vi "Traverse_Space.vi"(9 "Show Panel?":bool, 10 "Traverse Setup":string) -> (3 "Error Comments":string)   [LabVIEW 2011]
doc: "This is an example of using features of the VI Server as a client. It shows how you might browse from one or more applications that may be exporting data from one or more data stations. \n\nThe example shows how to query a server for its list of exported VIs, how to get references to the VIs, and how call them with the Call By Reference function."
uses:
  Route mapping/Exclude_cluster.ctl
  Route mapping/Box_size.ctl
  Route mapping/Exclusion_type.ctl
  Controls/ok_button.ctl
  Globals/Constants_global.vi
  Route mapping/Route_mapping_global.vi
  Globals/Trav_pos_global.vi
panel:
  in  "Traverse space filename":u16(ring) items=["Default_Space_file.xls", "---Save As---"]
  in  "Traverse Name":u16(ring) items=["A_Tunnel"]
  out "Message":string
  in  "Cancel Button":bool
  in  "OK":T1
  in  "Entire Space":T2=[{"Max"=15001.0, "Min"=12000.0}, {"Max"=1000.0, "Min"=-1000.0}, {"Max"=700.0, "Min"=0.0}] {"Min" format="%#.1f"; "Max" format="%#.1f"}
  in  "Probe Volume":T2=[{"Max"=15.0, "Min"=-15.0}, {"Max"=250.0, "Min"=0.0}, {"Max"=15.0, "Min"=-15.0}] {"Min" format="%#.1f"; "Max" format="%#.1f"}
  in  "Exclude Array":T3[](array[typedef])=[{"Sizes"=[{"Max"=15000.0, "Min"=0.0}, {"Max"=1000.0, "Min"=-1000.0}, {"Max"=300.0, "Min"=0.0}], "Name"="Roughness Elements", "Exclude Type"=enum."Allow only vertical moves"}, {"Sizes"=[{"Max"=17000.0, "Min"=16000.0}, {"Max"=200.0, "Min"=-200.0}, {"Max"=-50.0, "Min"=-250.0}], "Name"="B204", "Exclude Type"=enum."Exclude completely"}] {"Sizes"."Min" format="%#.1f"; "Sizes"."Max" format="%#.1f"}
  # "Enter all coordinates assuming the Model Orientation is zero degrees"
  # "(Relative to measurement position)"
  # "X                           Y                          Z"
  # "X                           Y                          Z"
  # "(Relative to measurement position)"
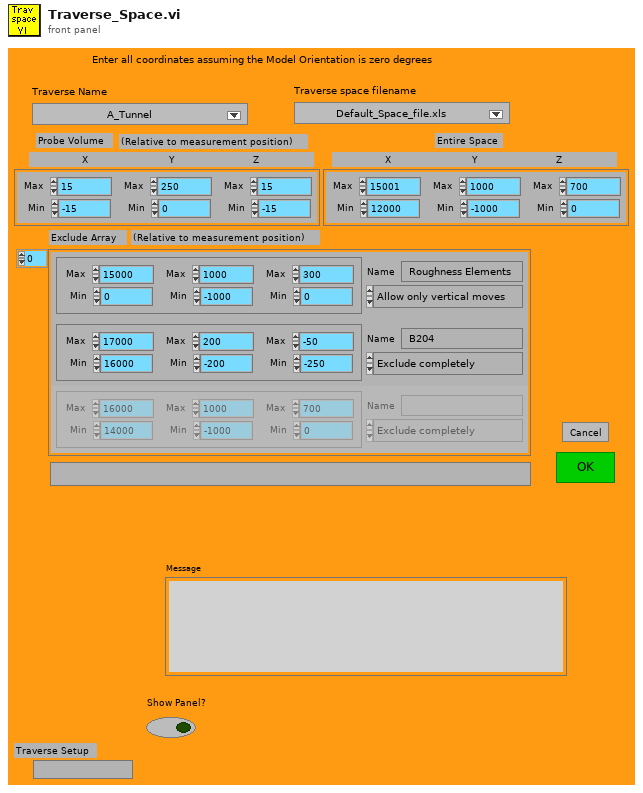
[diagram p1: front panel]
types:
  T1 = typedef "ok_button.ctl" = bool
  T2 = typedef "Box_size.ctl" = cluster{"Max":dbl, "Min":dbl}[]
  T3 = typedef "Exclude_cluster.ctl" = cluster{"Sizes":T2, "Name":string, "Exclude Type":T4}
  T4 = typedef "Exclusion_type.ctl" = enum16{"Exclude completely", "Allow only vertical moves"}
  T5 = enum16{"Load setup from excel file", "Save setup to excel file"}
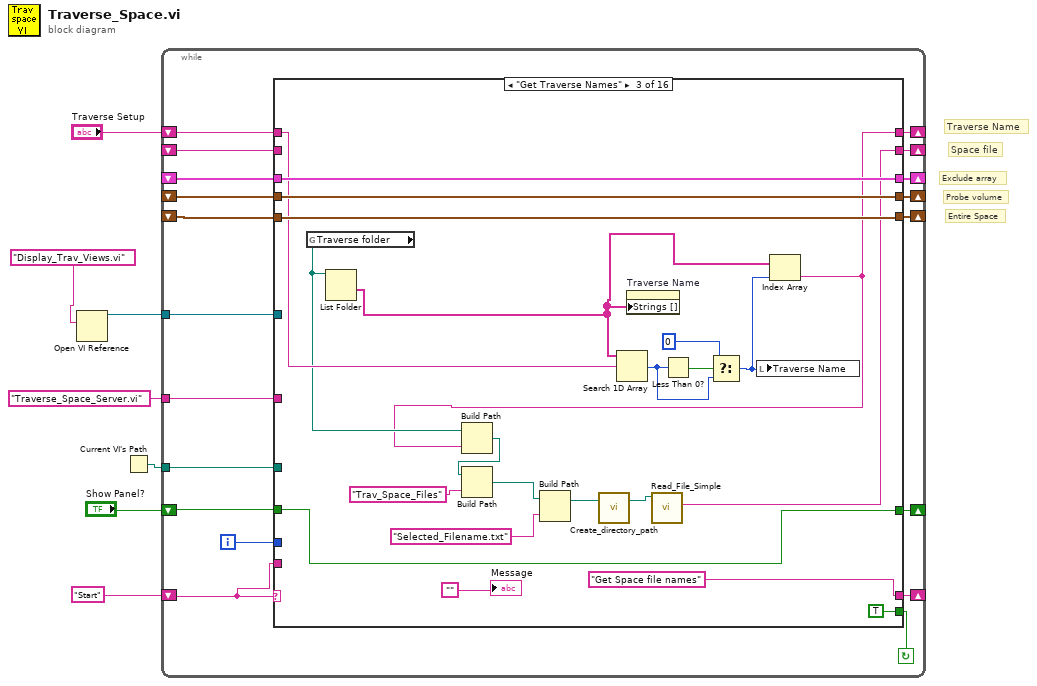
[diagram p0: block diagram]
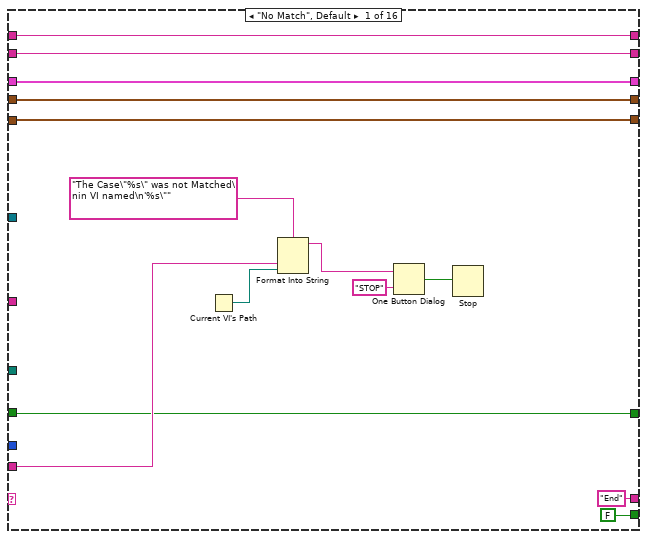
[diagram p2: hidden frame]
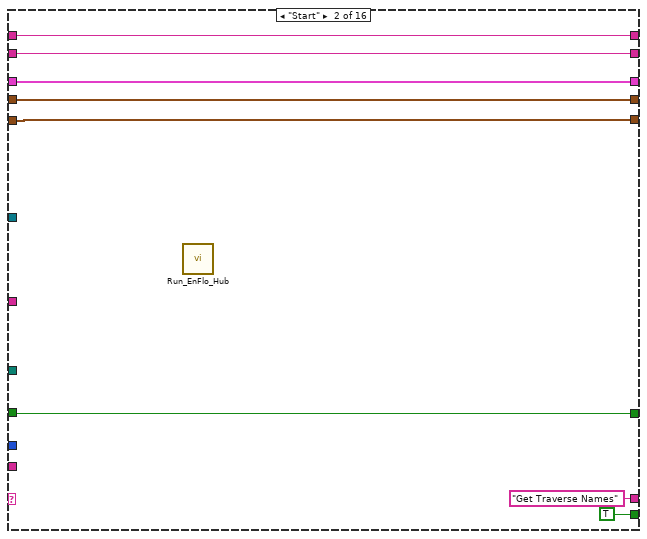
[diagram p3: hidden frame]
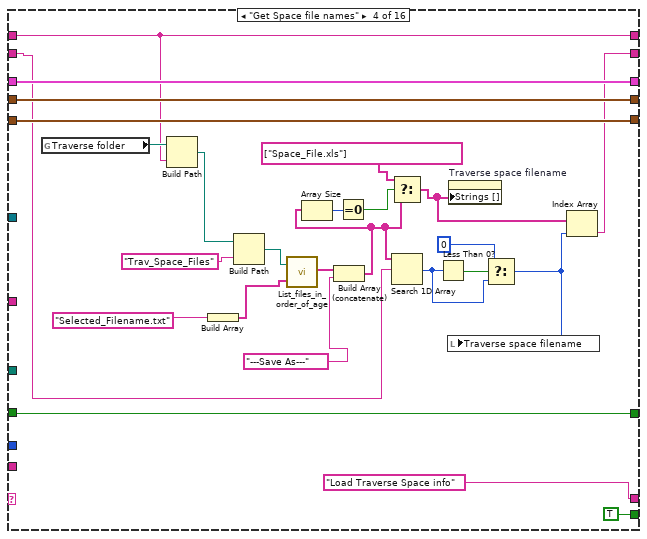
[diagram p4: hidden frame]
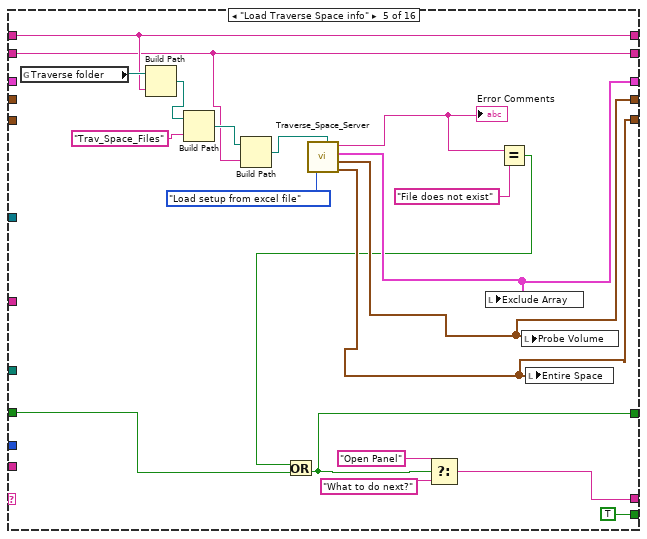
[diagram p5: hidden frame]
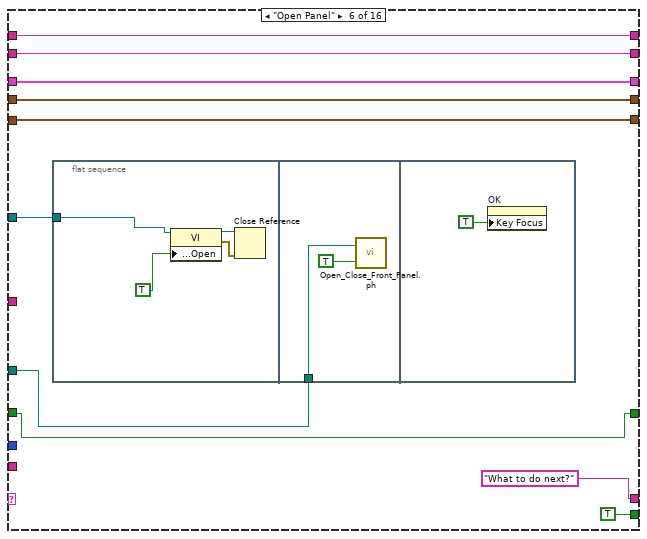
[diagram p6: hidden frame]
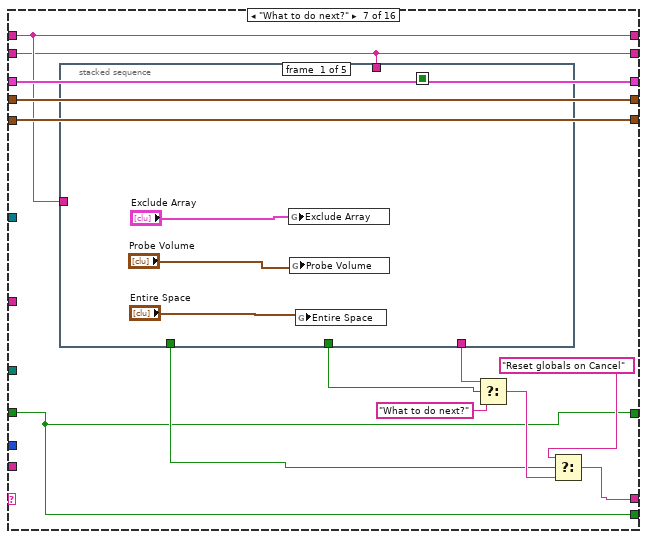
[diagram p7: hidden frame]
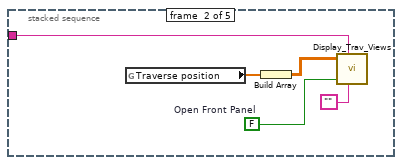
[diagram p8: hidden frame]
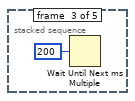
[diagram p9: hidden frame]
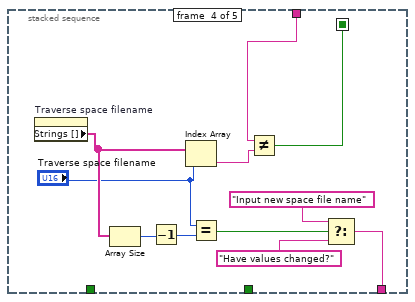
[diagram p10: hidden frame]
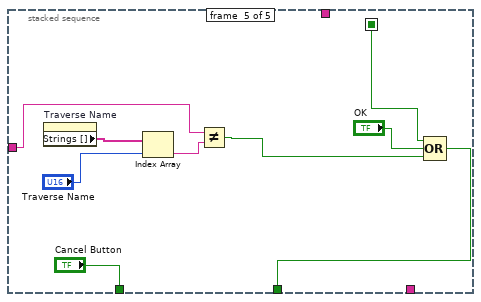
[diagram p11: hidden frame]
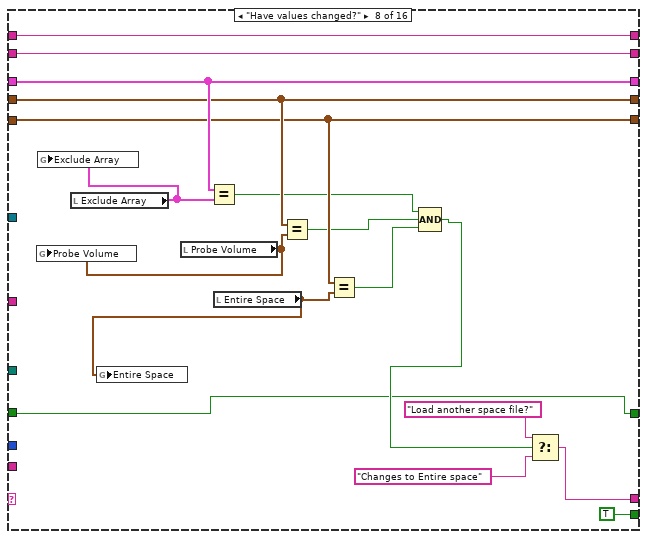
[diagram p12: hidden frame]
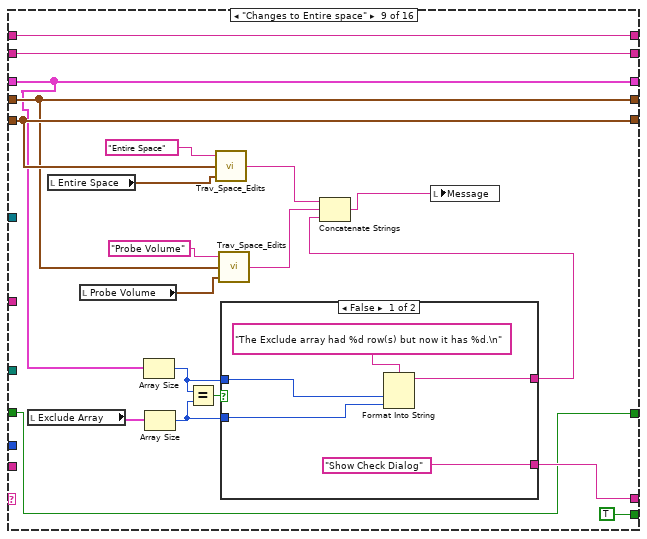
[diagram p13: hidden frame]
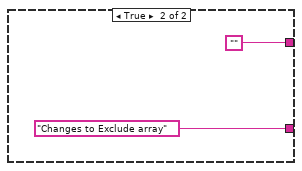
[diagram p14: hidden frame]
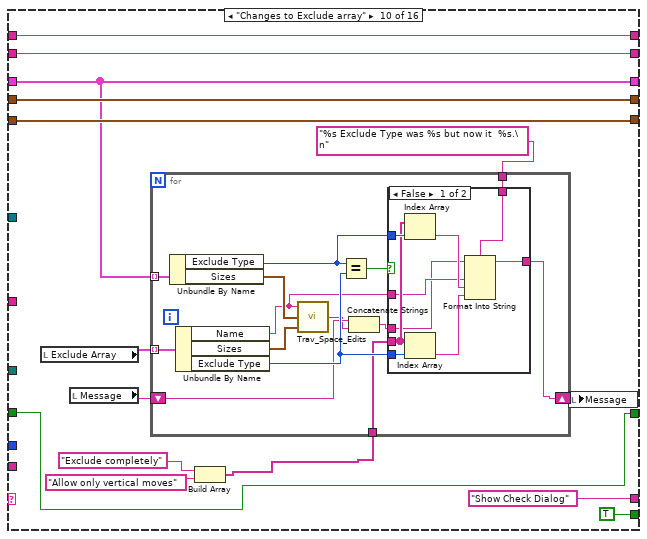
[diagram p15: hidden frame]
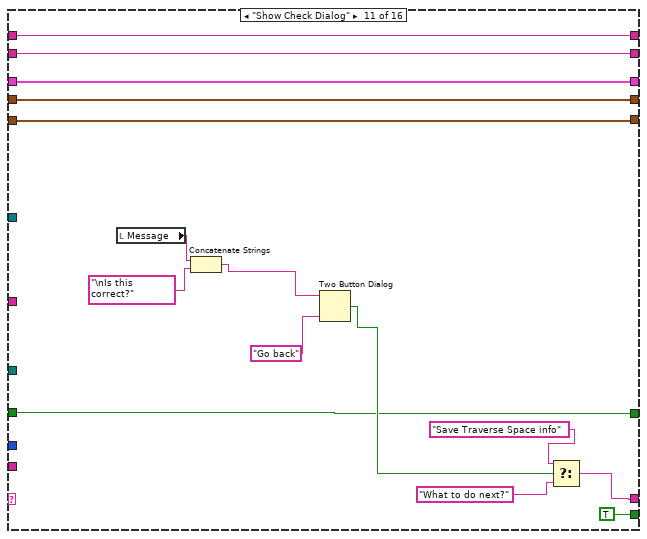
[diagram p17: hidden frame]
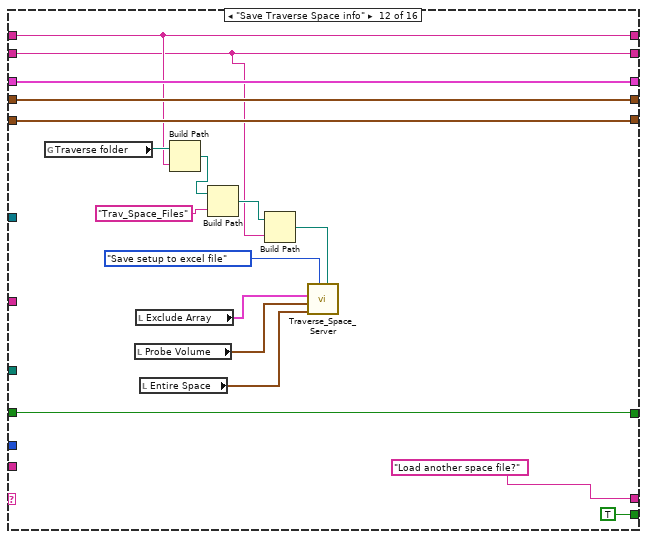
[diagram p18: hidden frame]
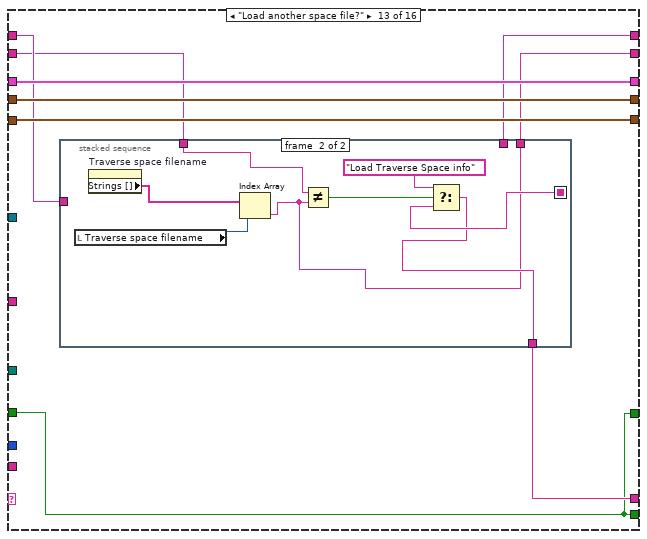
[diagram p19: hidden frame]
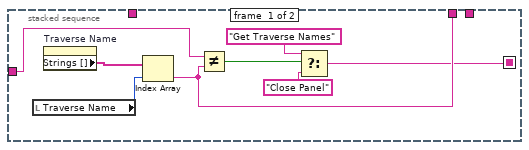
[diagram p20: hidden frame]
diagram:
  # "Traverse Name"
  # "Space file"
  # "Entire Space"
  # "Probe volume"
  # "Exclude array"
  n1 = Open VI Reference(vi path="Display_Trav_Views.vi") -> (vi reference=w1:refnum<vi>)  [unwired: 1 in, 5 out]
  n2 = Current VI's Path() -> (path=w5:path)
  n3 = while {
    tunnel: "Traverse_Space_Server.vi" ("VI name to run on server") -> [w24]
    shift-left: "Start" -> [w21]
    shift-right: [w23] -> _
    tunnel: w5 -> [w22]
    shift-right: [w20] -> _
    shift-left: _ -> [w17]
    shift-right: [w19] -> _
    shift-left: _ -> [w16]
    shift-right: [w18] -> _
    shift-left: _ -> [w15]
    shift-right: [w13] -> _
    shift-left: "Traverse Setup" -> [w11]
    shift-right: [w14] -> _
    shift-left: _ -> [w12]
    shift-right: [w9] -> _
    shift-left: "Show Panel?" -> [w10]
    tunnel: w1 -> [w8]
    i -> [w26]
    stop <- w25 continue-if-true
    n4 = case shown="\"Get Traverse Names\"" w21 {
      tunnel: w26 -> [_ _ _ _ _ _ _ _ _ _ _ _ _ _ _ _]
      tunnel: [FALSE ("status") TRUE ("status") TRUE ("status") TRUE ("status") TRUE ("status") TRUE ("status") w134 TRUE ("status") TRUE ("status") TRUE ("status") TRUE ("status") TRUE ("status") w291 w316 TRUE ("status") FALSE ("status")] -> w25
      tunnel: ["End" ("f") "Get Traverse Names" ("f") "Get Space file names" "Load Traverse Space info" w115 "What to do next?" w145 w182 w200 "Show Check Dialog" ("f") w263 "Load another space file?" w292 w317 "Close Panel" "End"] -> w23
      tunnel: w24 -> [_ _ _ _ _ _ _ _ _ _ _ _ _ _ _ _]
      tunnel: w10 -> [w27 w41 w49 w71 w99 w118 w134 w179 w193 w220 w259 w274 w291 w316 w340 w352]
      tunnel: w22 -> [_ _ _ _ _ w121 _ _ _ _ _ _ _ _ _ w366]
      tunnel: w21 -> [w35 _ _ _ _ _ _ _ _ _ _ _ _ _ _ _]
      tunnel: [w32 w48 w68 w94 w114 w124 w143 w192 w203 w230 w273 w288 w299 w327 w346 w365] -> w20
      tunnel: [w31 w47 w67 w93 w113 w123 w142 w191 w206 w232 w272 w287 w298 w326 w345 w364] -> w19
      tunnel: [w30 w46 w66 w92 w112 w122 w141 w190 w210 w233 w270 w286 w297 w325 w344 w363] -> w18
      tunnel: w17 -> [w32 w48 w68 w94 _ w124 w143 w192 w203 w230 w273 w288 w299 w327 w346 w365]
      tunnel: w16 -> [w31 w47 w67 w93 _ w123 w142 w191 w206 w232 w272 w287 w298 w326 w345 w364]
      tunnel: w15 -> [w30 w46 w66 w92 _ w122 w141 w190 w210 w233 w270 w286 w297 w325 w344 w363]
      tunnel: [w28 w42 w51 w77 w103 w119 w137 w180 w194 w221 w260 w276 w293 w320 w341 w353] -> w14
      tunnel: [w29 w43 w57 w76 w107 w120 w138 w181 w195 w222 w261 w277 w295 w324 w342 w358] -> w13
      tunnel: w12 -> [w28 w42 _ w75 w103 w119 w137 w180 w194 w221 w260 w276 w294 w319 w341 w353]
      tunnel: w11 -> [w29 w43 w60 w76 w107 w120 w138 w181 w195 w222 w261 w277 w296 w324 w342 w358]
      tunnel: [w27 w41 w49 w71 w97 w118 w134 w179 w193 w220 w259 w274 w291 w316 w340 w352] -> w9
      tunnel: w8 -> [_ _ _ _ _ w117 _ _ _ _ _ _ _ _ _ w348]
      frame "No Match", Default {
        n5 = Current VI's Path() -> (path=w40:path)
        n6 = Format Into String(format string="The Case\"%s\" was not Matched\nin VI named\n'%s\"" ("Format String"), w35, w40) -> (resulting string=w37:string)  [unwired: 2 in, 1 out]
        n7 = One Button Dialog(message=w37, button name ("OK")="STOP") -> (true=w39:bool)
        n8 = Stop(stop? (T)=w39) -> ()
      }
      frame "Start" {
        n9 = call "Run_EnFlo_Hub.vi"() -> ()  [unwired: 8 out]
      }
      frame "Get Traverse Names" {
        n10 = global read "Constants_global.vi" "Traverse folder"() -> (w58:path)
        n11 = List Folder(path=w58) -> (folder names=w50:string[])  [unwired: 1 in, 5 out]
        n12 = Search 1D Array(1D array=w50, element=w60) -> (index of element=w63:i32)  [unwired: 1 out]
        n13 = property on="Traverse Name" class="Ring (strict)"("Strings []"=w50) -> ()  [unwired: 2 in, 2 out]
        n14 = Less Than 0?(x=w63) -> (x < 0?=w64:bool)
        n15 = Select(t=0, s=w64, f=w63) -> (s? t:f=w61:i32)
        n16 = local write "Traverse Name"(w61) -> ()
        n17 = Index Array(array=w50, index=w61) -> (element=w57:string)
        n18 = Build Path(base path=w58, name or relative path=w57) -> (appended path=w56:path)
        n19 = Build Path(base path=w56, name or relative path="Trav_Space_Files" ("Substring")) -> (appended path=w55:path)
        n20 = Build Path(base path=w55, name or relative path="Selected_Filename.txt" ("Substring")) -> (appended path=w52:path)
        n21 = call "Create_directory_path.vi"("Path name"=w52) -> ("Path name Out"=w53:path)  [unwired: 1 in, 1 out]
        n22 = call "Read_File_Simple.vi"("Filename"=w53) -> ("string"=w51:string)  [unwired: 2 in, 7 out]
        "Message" <- ""
      }
      frame "Get Space file names" {
        n23 = global read "Constants_global.vi" "Traverse folder"() -> (w88:path)
        n24 = Build Path(base path=w88, name or relative path=w76) -> (appended path=w86:path)
        n25 = Build Array("Selected_Filename.txt" ("Substring")) -> (w85:string[])
        n26 = Build Path(base path=w86, name or relative path="Trav_Space_Files" ("Substring")) -> (appended path=w78:path)
        n27 = call "List_files_in_order_of_age.vi"("Files to Hide"=w85, "Folder"=w78) -> ("file names"=w74:string[])
        n28 = Build Array (concatenate)(w74, "---Save As---") -> (w73:string[])
        n29 = Array Size(array=w73) -> (size(s)=w83:i32)
        n30 = Equal To 0?(x=w83) -> (x = 0?=w82:bool)
        n31 = Select(t=string[] ["Space_File.xls"] ("appended array"), s=w82, f=w73) -> (s? t:f=w80:string[])
        n32 = Search 1D Array(1D array=w73, element=w75) -> (index of element=w90:i32)  [unwired: 1 out]
        n33 = Less Than 0?(x=w90) -> (x < 0?=w91:bool)
        n34 = property on="Traverse space filename" class="Ring (strict)"("Strings []"=w80) -> ()  [unwired: 2 in, 2 out]
        n35 = Select(t=0, s=w91, f=w90) -> (s? t:f=w79:i32)
        n36 = local write "Traverse space filename"(w79) -> ()
        n37 = Index Array(array=w80, index=w79) -> (element=w77:string)
      }
      frame "Load Traverse Space info" {
        n38 = global read "Constants_global.vi" "Traverse folder"() -> (w108:path)
        n39 = Build Path(base path=w108, name or relative path=w107) -> (appended path=w105:path)
        n40 = Build Path(base path=w105, name or relative path="Trav_Space_Files" ("Substring")) -> (appended path=w104:path)
        n41 = Build Path(base path=w104, name or relative path=w103) -> (appended path=w102:path)
        n42 = call "Traverse_Space_Server.vi"("Space File"=w102, "Mode"=T5."Load setup from excel file") -> ("Entire Space Out"=w112:T2, "Probe Volume Out"=w113:T2, "Exclude Array Out"=w114:T3[], "Error Comments"=w100:string)  [unwired: 5 in]
        "Error Comments" <- w100
        n43 = local write "Exclude Array"(w114) -> ()
        n44 = Equal?(x=w100, y="File does not exist") -> (x = y?=w98:bool)
        n45 = Or(x=w98, y=w99) -> (x .or. y?=w97:bool)
        n46 = Select(t="Open Panel", s=w97, f="What to do next?") -> (s? t:f=w115:string)
        n47 = local write "Probe Volume"(w113) -> ()
        n48 = local write "Entire Space"(w112) -> ()
      }
      frame "Open Panel" {
        n49 = flat-sequence {
          tunnel: w117 -> [w127]
          tunnel: w121 -> [w131]
          frame #0 {
            n50 = property class="VI"(reference=w127, "Front Panel Window:Open"=TRUE) -> (reference out=w129:refnum<vi>, error out=w128:errorcluster)  [unwired: 1 in]
            n51 = Close Reference(reference=w129, error in (no error)=w128) -> ()  [unwired: 1 out]
          }
          frame #1 {
            n52 = call "Open_Close_Front_Panel.ph.vi"("Front Panel Window:Open"=TRUE, "VI path"=w131) -> ()  [unwired: 2 out]
          }
          frame #2 {
            n53 = property on="OK" class="Bool"("Key Focus"=TRUE) -> ()  [unwired: 2 in, 2 out]
          }
        }
      }
      frame "What to do next?" {
        n54 = stacked-sequence {
          seq-local: [_ _ _ w160 _] -> [_ _ _ _ w167]
          tunnel: w138 -> [_ w150 _ _ w172]
          tunnel: [_ _ _ _ w168] -> w140
          tunnel: [_ _ _ _ "Cancel Button"] -> w139
          tunnel: w137 -> [_ _ _ w161 _]
          tunnel: [_ _ _ w157 _] -> w135
          frame #0 {
            n55 = global write "Route_mapping_global.vi" "Exclude Array"("Exclude Array") -> ()
            n56 = global write "Route_mapping_global.vi" "Probe Volume"("Probe Volume") -> ()
            n57 = global write "Route_mapping_global.vi" "Entire Space"("Entire Space") -> ()
          }
          frame #1 {
            w151 = FALSE  # Open Front Panel
            n58 = global read "Trav_pos_global.vi" "Traverse position"() -> (w152:dbl[])
            n59 = Build Array(w152) -> (w153:dbl[][])
            n60 = call "Display_Trav_Views.vi"("Current Probe Position"=w153, "Traverse Name"=w150, "Open Front Panel"=w151, "Error Comments"="") -> ()  [unwired: 3 in, 4 out]
          }
          frame #2 {
            n61 = Wait Until Next ms Multiple(millisecond multiple=u32 200) -> ()  [unwired: 1 out]
          }
          frame #3 {
            n62 = property on="Traverse space filename" class="Ring (strict)"() -> ("Strings []"=w163:string[])  [unwired: 2 in, 2 out]
            n63 = Array Size(array=w163) -> (size(s)=w165:i32)
            n64 = Decrement(x=w165) -> (x-1=w164:i32)
            n65 = Index Array(array=w163, index="Traverse space filename") -> (element=w166:string)
            n66 = Equal?(x="Traverse space filename", y=w164) -> (x = y?=w159:bool)
            n67 = Not Equal?(x=w161, y=w166) -> (x != y?=w160:bool)
            n68 = Select(t="Input new space file name" ("f"), s=w159, f="Have values changed?") -> (s? t:f=w157:string)
          }
          frame #4 {
            n69 = property on="Traverse Name" class="Ring (strict)"() -> ("Strings []"=w173:string[])  [unwired: 2 in, 2 out]
            n70 = Index Array(array=w173, index="Traverse Name") -> (element=w171:string)
            n71 = Not Equal?(x=w172, y=w171) -> (x != y?=w170:bool)
            n72 = Compound Arithmetic op=OR(w167, "OK", w170) -> (w168:T1)
          }
        }
        n73 = Select(t=w135, s=w140, f="What to do next?") -> (s? t:f=w146:string)
        n74 = Select(t="Reset globals on Cancel", s=w139, f=w146) -> (s? t:f=w145:string)
      }
      frame "Have values changed?" {
        n75 = local read "Exclude Array"() -> (w178:T3[])
        n76 = global write "Route_mapping_global.vi" "Exclude Array"(w178) -> ()
        n77 = local read "Probe Volume"() -> (w177:T2)
        n78 = global write "Route_mapping_global.vi" "Probe Volume"(w177) -> ()
        n79 = Equal?(x=w192, y=w178) -> (x = y?=w189:bool)
        n80 = local read "Entire Space"() -> (w176:T2)
        n81 = global write "Route_mapping_global.vi" "Entire Space"(w176) -> ()
        n82 = Equal?(x=w191, y=w177) -> (x = y?=w188:bool)
        n83 = Equal?(x=w190, y=w176) -> (x = y?=w187:bool)
        n84 = Compound Arithmetic op=AND(w189, w188, w187) -> (w185:bool)
        n85 = Select(t="Load another space file?", s=w185, f="Changes to Entire space") -> (s? t:f=w182:string)
      }
      frame "Changes to Entire space" {
        n86 = local read "Exclude Array"() -> (w202:T3[])
        n87 = local read "Entire Space"() -> (w209:T2)
        n88 = local read "Probe Volume"() -> (w207:T2)
        n89 = Array Size(array=w203) -> (size(s)=w199:i32)
        n90 = Array Size(array=w202) -> (size(s)=w198:i32)
        n91 = Equal?(x=w199, y=w198) -> (x = y?=w201:bool)
        n92 = call "Trav_Space_Edits.vi"("New"=w209, "Original"=w210, "Row Name"="Entire Space") -> ("Changes"=w205:string)
        n93 = call "Trav_Space_Edits.vi"("New"=w207, "Original"=w206, "Row Name"="Probe Volume") -> ("Changes"=w204:string)
        n94 = case shown="False" w201 {
          tunnel: ["Show Check Dialog" ("f") "Changes to Exclude array" ("f")] -> w200
          tunnel: w199 -> [w216 _]
          tunnel: w198 -> [w215 _]
          tunnel: [w213 ""] -> w197
          frame False {
            n95 = Format Into String(format string="The Exclude array had %d row(s) but now it has %d.\n", w216, w215) -> (resulting string=w213:string)  [unwired: 2 in, 1 out]
          }
          frame True {
          }
        }
        n96 = Concatenate Strings(w205, w204, w197) -> (w196:string)
        n97 = local write "Message"(w196) -> ()
      }
      frame "Changes to Exclude array" {
        n98 = local read "Exclude Array"() -> (w231:T3[])
        n99 = local read "Message"() -> (w224:string)
        n100 = Build Array("Exclude completely", "Allow only vertical moves") -> (w227:string[])
        n101 = for {
          tunnel: w230 -> [w246] mode=indexing
          tunnel: w231 -> [w248] mode=indexing
          shift-right: [w238] -> w225
          shift-left: w224 -> [w236]
          tunnel: w227 -> [w241]
          tunnel: "%s Exclude Type was %s but now it  %s.\n" ("format string") -> [w240]
          n102 = Unbundle By Name(w246) -> ("Exclude Type"=w242:T4, "Sizes"=w245:T2)
          n103 = Unbundle By Name(w248) -> ("Name"=w239:string, "Sizes"=w247:T2, "Exclude Type"=w243:T4)
          n104 = call "Trav_Space_Edits.vi"("New"=w247, "Original"=w245, "Row Name"=w239) -> ("Changes"=w235:string)
          n105 = Equal?(x=w242, y=w243) -> (x = y?=w244:bool)
          n106 = Concatenate Strings(w236, w235) -> (w237:string)
          n107 = case shown="False" w244 {
            tunnel: w243 -> [w257 _]
            tunnel: w242 -> [w256 _]
            tunnel: w241 -> [w255 _]
            tunnel: w240 -> [w252 _]
            tunnel: w239 -> [w251 _]
            tunnel: w237 -> [w250 w258]
            tunnel: [w249 w258] -> w238
            frame False {
              n108 = Index Array(array=w255, index=w256) -> (element=w253:string)
              n109 = Index Array(array=w255, index=w257) -> (element=w254:string)
              n110 = Format Into String(format string=w252, initial string=w250, w251, w253, w254) -> (resulting string=w249:string)  [unwired: 1 in, 1 out]
            }
            frame True {
            }
          }
        }
        n111 = local write "Message"(w225) -> ()
      }
      frame "Show Check Dialog" {
        n112 = local read "Message"() -> (w269:string)
        n113 = Concatenate Strings(w269, "\nIs this correct?") -> (w268:string)
        n114 = Two Button Dialog(message=w268, 1:"Go back" ("F button name (\"Cancel\")")) -> (T button?=w265:bool)  [unwired: 1 out]
        n115 = Select(t="Save Traverse Space info", s=w265, f="What to do next?") -> (s? t:f=w263:string)
      }
      frame "Save Traverse Space info" {
        n116 = global read "Constants_global.vi" "Traverse folder"() -> (w281:path)
        n117 = local read "Probe Volume"() -> (w283:T2)
        n118 = local read "Exclude Array"() -> (w284:T3[])
        n119 = local read "Entire Space"() -> (w282:T2)
        n120 = Build Path(base path=w281, name or relative path=w277) -> (appended path=w279:path)
        n121 = Build Path(base path=w279, name or relative path="Trav_Space_Files" ("Substring")) -> (appended path=w278:path)
        n122 = Build Path(base path=w278, name or relative path=w276) -> (appended path=w275:path)
        n123 = call "Traverse_Space_Server.vi"("Space File"=w275, "Mode"=T5."Save setup to excel file", "Entire Space"=w282, "Probe Volume"=w283, "Exclude Array"=w284) -> ()  [unwired: 2 in, 4 out]
      }
      frame "Load another space file?" {
        n124 = stacked-sequence {
          seq-local: [w301 _] -> [_ w313]
          tunnel: w296 -> [w306 _]
          tunnel: [w302 _] -> w295
          tunnel: [_ w310] -> w292
          tunnel: w294 -> [_ w308]
          tunnel: [_ w309] -> w293
          frame #0 {
            n125 = local read "Traverse Name"() -> (w300:u16)
            n126 = property on="Traverse Name" class="Ring (strict)"() -> ("Strings []"=w307:string[])  [unwired: 2 in, 2 out]
            n127 = Index Array(array=w307, index=w300) -> (element=w302:string)
            n128 = Not Equal?(x=w306, y=w302) -> (x != y?=w305:bool)
            n129 = Select(t="Get Traverse Names" ("f"), s=w305, f="Close Panel") -> (s? t:f=w301:string)
          }
          frame #1 {
            n130 = local read "Traverse space filename"() -> (w311:u16)
            n131 = property on="Traverse space filename" class="Ring (strict)"() -> ("Strings []"=w312:string[])  [unwired: 2 in, 2 out]
            n132 = Index Array(array=w312, index=w311) -> (element=w309:string)
            n133 = Not Equal?(x=w308, y=w309) -> (x != y?=w314:bool)
            n134 = Select(t="Load Traverse Space info" ("f"), s=w314, f=w313) -> (s? t:f=w310:string)
          }
        }
      }
      frame "Input new space file name" {
        n135 = property on="Traverse space filename" class="Ring (strict)"() -> ("Strings []"=w318:string[])  [unwired: 2 in, 2 out]
        n136 = call "Input_String_Dialog.vi"("Message to user"="Please Enter a new  space file name") -> ("Ok Out"=w321:bool, "Output string"=w322:string)  [unwired: 1 in]
        n137 = case shown="True" w321 {
          tunnel: w322 -> [_ w335]
          tunnel: [w329 w330] -> w320
          tunnel: w319 -> [w329 _]
          tunnel: w318 -> [_ w331]
          tunnel: ["What to do next?" ("f") "Save Traverse Space info" ("f")] -> w317
          frame False {
          }
          frame True {
            n138 = call "Fast_string_Replace.vi"("Replace match with:"="_", "Input String"=w335, "regular expression"=" ") -> ("Output String"=w336:string)  [unwired: 2 out]
            n139 = local write "Traverse space filename"(0) -> ()
            n140 = call "Add_filename_suffix.vi"("Filename"=w336, "Suffix to add"=".xls") -> ("Filename out"=w330:string)  [unwired: 3 out]
            n141 = Build Array (concatenate)(w330, w331) -> (w334:string[])
            n142 = property on="Traverse space filename" class="Ring (strict)"("Strings []"=w334) -> ()  [unwired: 2 in, 2 out]
          }
        }
      }
      frame "Reset globals on Cancel" {
        n143 = global write "Route_mapping_global.vi" "Entire Space"(w344) -> ()
        n144 = global write "Route_mapping_global.vi" "Probe Volume"(w345) -> ()
        n145 = global write "Route_mapping_global.vi" "Exclude Array"(w346) -> ()
      }
      frame "Close Panel" {
        w356 = FALSE  # append to file? (new file:F)
        w357 = FALSE  # advisory dialog? (display:T)
        n146 = global read "Constants_global.vi" "Traverse folder"() -> (w362:path)
        n147 = call "Open_Close_Front_Panel.ph.vi"("Front Panel Window:Open"=FALSE, "VI path"=w366) -> ()  [unwired: 2 out]
        n148 = Build Path(base path=w362, name or relative path=w358) -> (appended path=w360:path)
        n149 = Build Path(base path=w360, name or relative path="Trav_Space_Files" ("Substring")) -> (appended path=w359:path)
        n150 = Build Path(base path=w359, name or relative path="Selected_Filename.txt" ("Substring")) -> (appended path=w354:path)
        n151 = property class="VI"(reference=w348, "Front Panel Window:Open"=FALSE) -> (reference out=w350:refnum<vi>, error out=w349:errorcluster)  [unwired: 1 in]
        n152 = Close Reference(reference=w350, error in (no error)=w349) -> ()  [unwired: 1 out]
        n153 = call "Write_Characters_To_File.vi"("file path (dialog if empty)"=w354, "advisory dialog? (display:T)"=w357, "character string"=w353, "append to file? (new file:F)"=w356) -> ()  [unwired: 1 in, 4 out]
      }
    }
  }
